vi "Change Single Number's Digits.vi"(9 "precision (6)":i16=2, 11 "number":dbl) -> (2 "F-format string":string, 3 "number 2":dbl)   [LabVIEW 2021]
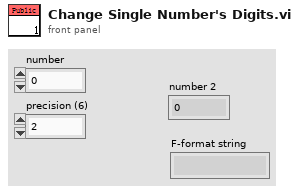
[diagram p1: front panel]
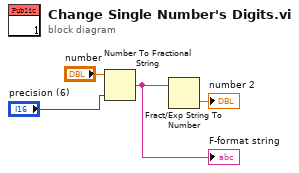
[diagram p0: block diagram]
diagram:
  n1 = Number To Fractional String(number="number", precision (6)="precision (6)") -> (F-format string=w4:string)  [unwired: 2 in]
  "F-format string" <- w4
  n2 = Fract/Exp String To Number(string=w4) -> (number=→"number 2":dbl)  [unwired: 3 in, 1 out]
